vi "VHT LTF 80MHz LUT.vi"(9 "frequency offset index":fxp<+/-,9,9>) -> (1 "VHT LTF symbol":T1)   [LabVIEW 2020]
uses:
  <vilib>/rvi/Memory/Memory_Emulation/nirvimemoryFastEmulation.vi
  <vilib>/rvi/Memory/Memory_Emulation/nirvimemoryEmulation.vi
  <vilib>/rvi/Emulation/niFpgaEmulationIsFPGAContextNoSignature.vi
  <vilib>/rvi/DataTransferAndStorage/Container/Common/niFpgaContainerGetUniqueNameForEmu.vi
  <vilib>/rvi/Emulation/niFpgaProcessEmulError.vi
  <vilib>/rvi/Emulation/niFpgaSctlEmulationGetInTimedLoop.vi
  <vilib>/rvi/errors/nirviReportUnexpectedCaseInternalError (U32).vi
  <vilib>/rvi/DataTransferAndStorage/Container/XNode/niFpgaContainer.xnode
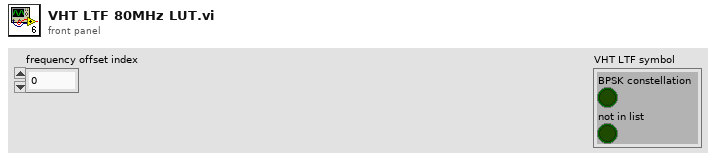
[diagram p1: front panel]
types:
  T1 = cluster{"BPSK constellation":bool, "not in list":bool}
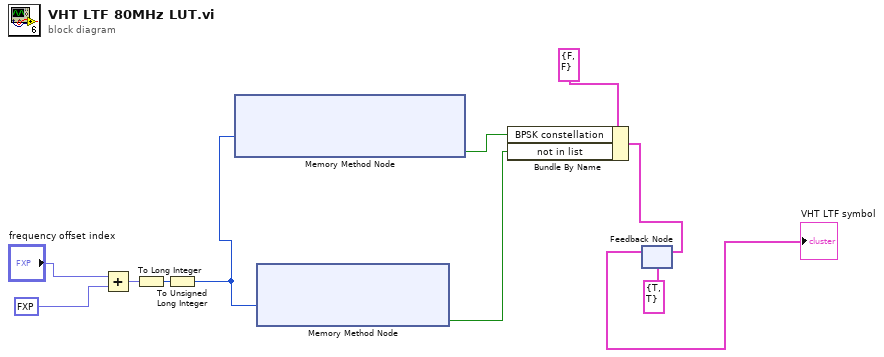
[diagram p0: block diagram]
diagram:
  n1 = Add(x="frequency offset index", y=fxp<+/-,9,9> 122.0) -> (x+y=w9:fxp<+/-,10,10>)
  n2 = To Long Integer(number=w9) -> (32bit integer=w8:i32)
  n3 = To Unsigned Long Integer(number=w8) -> (unsigned 32bit integer=w1:u32)
  n4 = xnode ("Memory Method Node")("Address"=w1) -> ("Data"=w3:bool)  [unwired: 1 in, 1 out]
  n5 = xnode ("Memory Method Node")("Address"=w1) -> ("Data"=w4:bool)  [unwired: 1 in, 1 out]
  n6 = Bundle By Name(cluster=T1 {"BPSK constellation"=FALSE, "not in list"=FALSE} ("Data"), "BPSK constellation"=w3, "not in list"=w4) -> (w2:T1)
  n7 = feedback #1(T1 {"BPSK constellation"=TRUE, "not in list"=TRUE} ("Data")) -> (→"VHT LTF symbol":T1)
  n8 = feedback-in #1(w2) -> ()
